vi "Constants.vi"() -> ()   [LabVIEW 2015, in "SLSC Module Template Shared.lvlib"]
doc: "Use this Global VI to access the GUIDs assigned to the page resources of the Custom Device."
uses:
  SLSC Module Template Shared.lvlib
panel:
  in  "Tab Control 2":T1(tab)=enum."Constants"
  in  "GUID EnableDisable Page":string="ab216e3e-ce56-4302-be76-5c073e8fefd9"
  in  "GUID Command Page":string="f13a2c78-8202-4aa2-888c-ebaa2cbdbf5d"
  in  "GUID Status  Page":string="91b8c77a-ac34-4100-a73c-37ebc6c9bffa"
  in  "GUID Outgoing Page":string="299fe32d-58d0-4147-8dde-bd157b2137cb"
  in  "GUID Incoming Page":string="44e24b3c-aef9-4263-8a05-733641b3eafe"
  in  "GUID Main Page":string="356fdb93-a7c7-48c3-9226-4c388c9f88c0"
  in  "GUID Channel Interface":string="9d7fe8e5-79ce-429b-943b-88e648e066ff"
  in  "CHM File Name":string="SLSC Module Addon.chm"
  in  "Channel Interface Name":string="Channel Interface"
  in  "Module.Name":string="SLSC Module Template Custom Device"
  in  "product.Num":i32=1
  in  "vendor.Num":i32=1
  in  "CD Version":string="1.0.0"
  in  "Command Channel":string="Commands"
  in  "Status Channel":string="Status"
  in  "Outgoing Channel":string="Outgoing"
  in  "Incoming Channel":string="Incoming"
  in  "SLSCChannelPath":string="SLSCChannelPath"
  in  "PropertyNames":string="PropertyNames"
  in  "Page Configuration Settings":string="Page Configuration Settings"
  in  "Compiled.Settings":string="Compiled.Settings"
  in  "productNum":string="productNum"
  in  "vendorNum":string="vendorNum"
  in  "Slot CD Processor Affinity":string="Slot CD Processor Affinity"
  in  "SLSC Root CD Version":string="SLSC Root CD Version"
  in  "SLSC Plug-in Paths":string="SLSC Plug-in Paths"
  in  "SLSC Plug-in GUIDs":string="SLSC Plug-in GUIDs"
  in  "SLSC Plug-in Names":string="SLSC Plug-in Names"
  in  "ModuleName":string="ModuleName"
  in  "Module Number":string="Slot #"
  in  "Chassis #":string="Chassis #"
  in  "Chassis IP Address":string="Chassis IP Address"
  in  "SlotX.Property":string="Slot %d.%s"
  in  "Slot CD Name Format":string="Slot %d (%s)"
  in  "Property.Property":string="%s.%s"
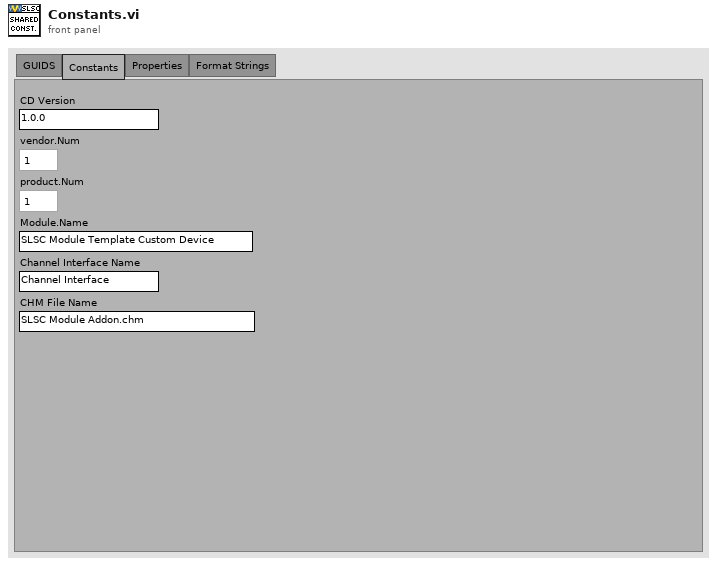
[diagram p1: front panel]
types:
  T1 = enum32{"GUIDS", "Constants", "Properties", "Format Strings"}
diagram:
